vi "thcd401_rezero.vi"(7 "CH":enum16{"", "1", "2", "3", "4"}(ring), 8 "error in":errorcluster, 11 "conn_id_in":refnum<k5>) -> (0 "error out":errorcluster, 3 "conn_id_out":refnum<k5>, 4 "status":bool)   [LabVIEW 2019]
panel:
  out "query":string
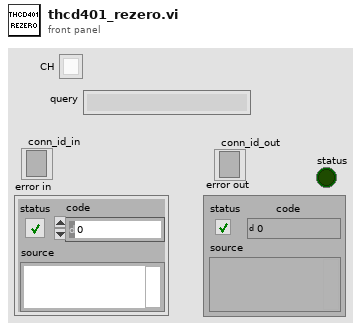
[diagram p1: front panel]
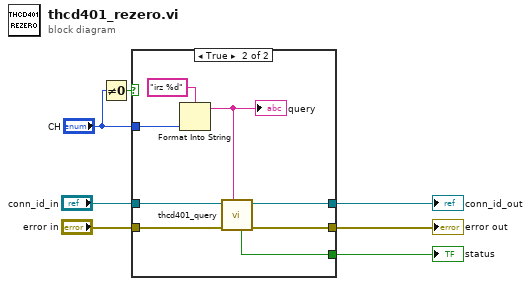
[diagram p0: block diagram]
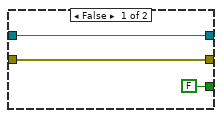
[diagram p2: hidden frame]
diagram:
  n1 = Not Equal To 0?(x="CH") -> (x != 0?=w2:bool)
  n2 = case shown="True" w2 {
    tunnel: "error in" -> [w9 w18]
    tunnel: [w10 w17] -> w6
    tunnel: "conn_id_in" -> [w10 w16]
    tunnel: [w9 w15] -> w4
    tunnel: [FALSE ("status") w14] -> w3
    tunnel: "CH" -> [_ w11]
    frame False {
    }
    frame True {
      n3 = Format Into String(format string="irz %d", w11) -> (resulting string=w12:string)  [unwired: 2 in, 1 out]
      "query" <- w12
      n4 = call "thcd401_query.vi"("command"=w12, "error in"=w18, "conn_id_in"=w16) -> ("error out"=w15:errorcluster, "conn_id_out"=w17:refnum<k5>, "status"=w14:bool)  [unwired: 5 in, 1 out]
    }
  }
  "error out" <- w4
  "status" <- w3
  "conn_id_out" <- w6
